vi "Reverse 1D Array.vi"(7 "JSON Array":refnum<class "JSON Array.lvclass">) -> (8 "reversed JSON Array":refnum<class "JSON Array.lvclass">)   [LabVIEW 2016, in "LVJSON.lvlib" / "JSON Array.lvclass"]
doc: "Reverses the order of the elements in array, where array is of any type."
uses:
  JSON Array.lvclass
  JSON Array.lvclass/JSON Array.ctl
  JSON Datatype/JSON Null.lvclass
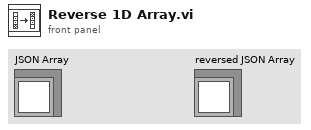
[diagram p1: front panel]
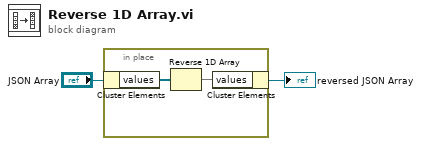
[diagram p0: block diagram]
diagram:
  n1 = in-place {
    n2 = in-place-cluster #1("JSON Array") -> ("values"=w4:refnum<class "JSON Null.lvclass">[])
    n3 = Reverse 1D Array(array=w4) -> (reversed array=w3:refnum<class "JSON Null.lvclass">[])
    n4 = in-place-cluster #1("values"=w3) -> (→"reversed JSON Array":refnum<class "JSON Array.lvclass">)
  }
